vi "Camber controller May 13 2016.vi"() -> ()   [LabVIEW 2014]
uses:
  Environmental Chamber LabVIEW and Instruments/Drivers and Software/keithley_24xx/Keithley 24XX/Keithley 24XX.lvlib
  Environmental Chamber LabVIEW and Instruments/Drivers and Software/keithley_6430/Keithley 6430/Keithley 6430.lvlib
  <vilib>/Instr/_visa.llb/VISA Configure Serial Port (Instr).vi
  <vilib>/Utility/file.llb/Write To Spreadsheet File (string).vi
  Environmental Chamber LabVIEW and Instruments/Drivers and Software/Keithley 2100 Series/Keithley 2100 Series.lvlib
  Environmental Chamber LabVIEW and Instruments/Drivers and Software/Keithley 2100 Series/Public/Configure/Configure 2 Wire Resistance.vi
  Environmental Chamber LabVIEW and Instruments/Drivers and Software/LabVIEW 8.2 Drivers/keithley_24xx/Keithley 24XX/Public/Data/Read (Single Point).vi
  Environmental Chamber LabVIEW and Instruments/Drivers and Software/keithley_6430/Keithley 6430/Public/Data/Read (Single Point).vi
  <vilib>/Utility/file.llb/Read From Spreadsheet File (string).vi
panel:
  out "Cluster":T1
  out "K-2100 (Ohm)":cluster{"Measurement":dbl}(graph)
  out "pressure chart":cluster{"pressure":dbl}(graph)
  out "K-6430 (Ohm)":cluster{"Measurement":dbl}(graph)
  out "K-2420 (Ohm)":cluster{"Resistance":sgl}(graph)
  in  "Data saving options":T2={"Save during sequence only"=TRUE, "Save now"=FALSE, "Stop program when sequence ends"=TRUE, "Delay between data points (s)"=0.0, "Experiment Notes"="", "Currently saving data"=FALSE, "Data file save path"=path ""} {"Delay between data points (s)" min=0.0 max=30.0 format="%#_13g"}
  in  "Set pressure parameters":T3={"valve % open"=100.0, "Desired pressure"=0.0, "Vapor sccm"=0.0, "Gas sccm"=0.0, "Valve"=enum."% Open", "Pressure Mode"=enum."Abs. pressure", "analyte partial pressure"=100.0} {"analyte partial pressure" min=0.0 max=100.0 step=5.0; "Gas sccm" min=0 max=200 step=5; "Vapor sccm" min=0 max=200 step=5; "Desired pressure" min=0.0 max=760.0 step=5.0; "valve % open" min=0.0 max=100.0 step=5.0 format="%#_2f"}
  out "Actual":T4 {"actual gas flow" format="%#_3g"; "Actual vapor flow" format="%#_3g"; "actual pressure" format="%#_3g"; "Valve position (%)" format="%#_2f"}
  out "arduino QCM plots":T5
  out "QCM Freq. (MHz)":T6 {"QCM1" format="%#_8g"; "QCM2" format="%#_8g"; "QCM3" format="%#_8g"; "QCM4" format="%#_8g"; "QCM5" format="%#_8g"; "QCM6" format="%#_8g"}
  in  "Sample names":T7={"QCM1"="aQCM2", "QCM2"="aQCM2", "QCM3"="aQCM3", "QCM4"="aQCM4", "QCM5"="aQCM5", "QCM6"="aQCM6", "SRS"="sample_SRS", "K-2420"="Keithley2420", "K-6430"="Keithley6430", "K-2100"="Keithley6430"}
  out "Sequence\npreview":cluster{dbl[], dbl[]}[](graph)
  in  "Gate time":u16(ring)=1 items=["0.1 seconds", "1.0 seconds", "10.0 seconds"]
  out "MHz":dbl format="%.6f"
  out "QCM plot":T8(graph)
  in  "User-defined\nsequence":string[][](table) caption="Create sequence"
  out "Sequence end time":string
  in  "Run Sequence":bool
  in  "Import sequence file":bool
  in  "Save sequence":bool
  in  "Clear sequence":bool
  in  "Turbo pump\nauto on":bool=TRUE caption="Turbo pump auto on"
  in  "stop":bool
  in  "Clear all charts":bool
  out "appended array":dbl[](array[numeric]) caption="atm\nTorr"
  in  "rapidox O2 Sensor":bool
  in  "setnag O2 Pump":bool
  in  "Baud Rate 2":i32(ring)=2 items=["2400", "4800", "9600", "19200", "38400", "57600", "115200"]
  in  "Com Port":i32(ring) items=["Com 1", "Com 2", "Com 3", "Com 4", "Com 5", "Com 6", "COM 7", "COM 8", "COM 9", "COM 10", "COM 11", "COM 12", "com 13", "COM 14"]
  in  "Com Port 2":i32(ring) items=["Com 1", "Com 2", "Com 3", "Com 4", "Com 5", "Com 6", "COM 7", "COM 8", "COM 9", "COM 10", "COM 11", "COM 12", "com 13", "COM 14"]
  out "Waveform Chart":cluster{dbl}(graph)
  out "O2 Concentration (PPM)":dbl
  out "Waveform Chart 6":cluster{dbl}(graph)
  # "Pressure Control"
  # "Gas/Vapor Sequence"
  # "SRS QCM"
  # "Currently Unused"
  # "100%"
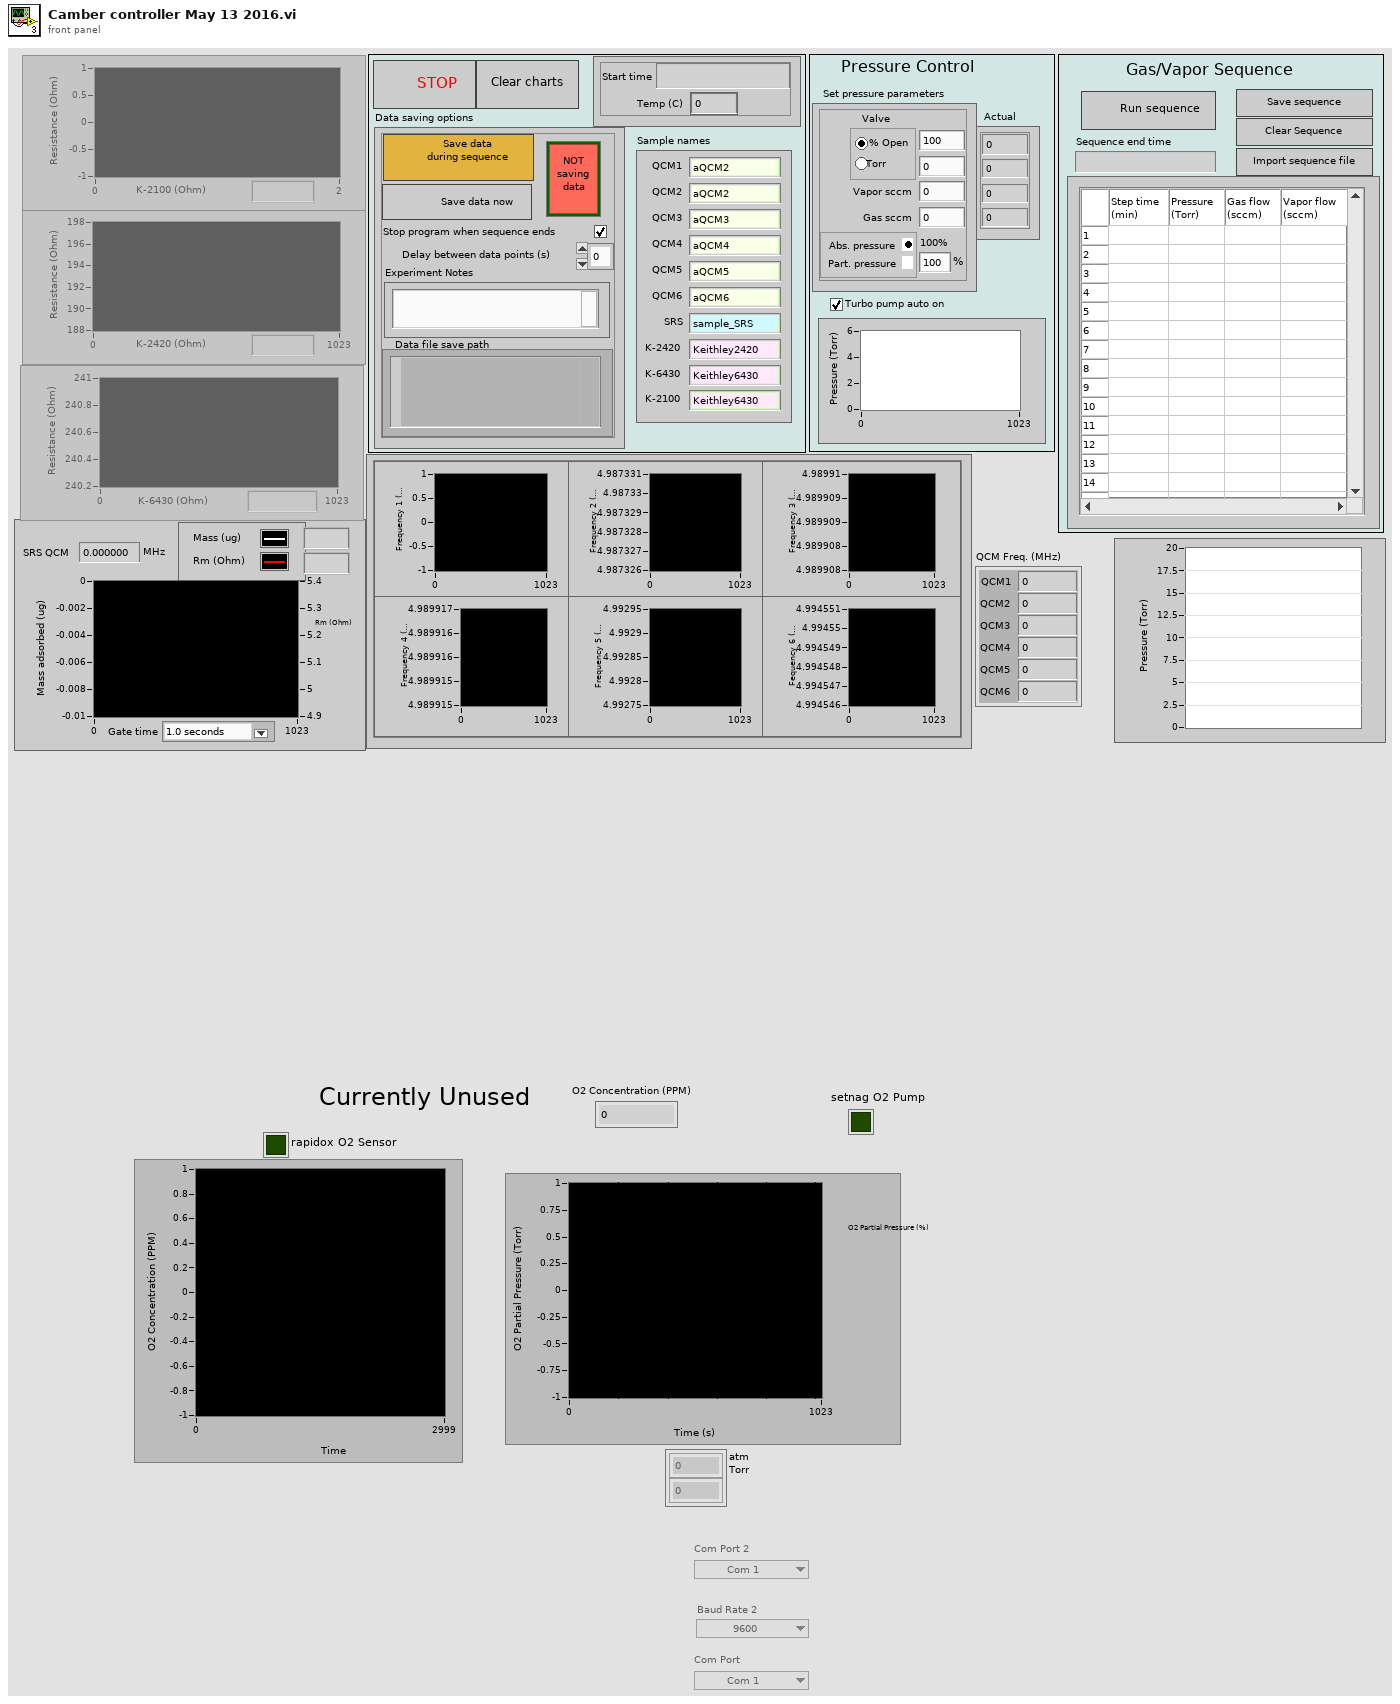
[diagram p1: front panel]
types:
  T1 = cluster{"State date/time":string, "Temp (C)":dbl}
  T2 = cluster{"Save during sequence only":bool, "Save now":bool, "Stop program when sequence ends":bool, "Delay between data points (s)":dbl, "Experiment Notes":string, "Currently saving data":bool, "Data file save path":path}
  T3 = cluster{"valve % open":dbl, "Desired pressure":dbl, "Vapor sccm":sgl, "Gas sccm":sgl, "Valve":enum32{"% Open", "Torr "}, "Pressure Mode":enum32{"Abs. pressure", " Part. pressure"}, "analyte partial pressure":dbl}
  T4 = cluster{"Valve position (%)":dbl, "actual pressure":dbl, "Actual vapor flow":dbl, "actual gas flow":dbl}
  T5 = cluster{"arduino qcm 1":dbl, "arduino qcm 2":dbl, "arduino qcm 3":dbl, "arduino qcm 4":dbl, "arduino qcm 5":dbl, "arduino qcm 6":dbl}
  T6 = cluster{"QCM1":dbl, "QCM2":dbl, "QCM3":dbl, "QCM4":dbl, "QCM5":dbl, "QCM6":dbl}
  T7 = cluster{"QCM1":string, "QCM2":string, "QCM3":string, "QCM4":string, "QCM5":string, "QCM6":string, "SRS":string, "K-2420":string, "K-6430":string, "K-2100":string}
  T8 = cluster{"Numeric Control":dbl, "Resistance out":dbl}
  T9 = enum16{"open", "open or create", "create or replace", "create", "open (read only)"}
  T10 = enum8{"Enabled", "Disabled", "Disabled and Grayed Out"}
  T11 = cluster{"task out":refnum<k21>, "error out":errorcluster, "task out":refnum<k21>, "error out":errorcluster, "task out":refnum<k21>, "error out":errorcluster, "VISA resource name":refnum<visa-resource-name>, "error out":errorcluster}
  T12 = cluster{"task out":refnum<k21>, "error out":errorcluster, "task out":refnum<k21>, "error out":errorcluster, "task out":refnum<k21>, "error out":errorcluster, "VISA resource name out":refnum<visa-resource-name>, "error out":errorcluster}
  T13 = enum16{"no parity", "odd parity", "even parity", "mark parity", "space parity"}
  T14 = cluster{bool, "VISA resource name":refnum<visa-resource-name>, "error out":errorcluster}
  T15 = cluster{bool, "VISA resource name out":refnum<visa-resource-name>, "error out":errorcluster}
  T16 = cluster{"Arduino 1":refnum<visa-resource-name>, "Arduino 2":refnum<visa-resource-name>, "Arduino 3":refnum<visa-resource-name>, "Arduino 4":refnum<visa-resource-name>, "Arduino 5":refnum<visa-resource-name>, "Arduino 6":refnum<visa-resource-name>}
  T17 = cluster{"VISA resource name out":refnum<visa-resource-name>, "error out":errorcluster, "VISA resource name out":refnum<visa-resource-name>, "error out":errorcluster, "VISA resource name out":refnum<visa-resource-name>, "error out":errorcluster, "VISA resource name out":refnum<visa-resource-name>, "error out":errorcluster, "VISA resource name out":refnum<visa-resource-name>, "error out":errorcluster, "VISA resource name out":refnum<visa-resource-name>, "error out":errorcluster}
  T18 = cluster{"f":dbl, "f":dbl, "f":dbl, "f":dbl, "f":dbl, "f":dbl}
  T19 = cluster{"String":string, "String":string, "String":string}
  T20 = cluster{"Boolean":bool, "VISA resource name out":refnum<visa-resource-name>, "error out":errorcluster}
  T21 = cluster{"Numeric Control":dbl, "Cluster":cluster{"Numeric Control":dbl}, "String":string, "error out":errorcluster}
  T22 = cluster{bool, "Turbo pump\nauto on":bool, "current  step # out":i32}
  T23 = cluster{"date/time string":string, "Temp (C)":dbl}
  T24 = cluster{"Present (s)":dbl, "Run Sequence":bool, "Set pressure parameters":cluster{"valve % open":dbl, "Desired pressure":dbl, "Vapor sccm":sgl, "Gas sccm":sgl, "Valve":enum32{"% Open", "Torr "}, "Pressure Mode":enum32{"Abs. pressure", " Part. pressure"}, "analyte partial pressure":dbl}, "sequence end time":timestamp}
  T25 = cluster{"f":dbl, "f":dbl, "f":dbl, "f":dbl, "f":dbl}[]
  T26 = cluster{"VISA Refnum out":refnum<visa-resource-name>, "error out":errorcluster, "VISA Refnum out":refnum<visa-resource-name>, "error out":errorcluster, "VISA Refnum out":refnum<visa-resource-name>, "error out":errorcluster, "VISA Refnum out":refnum<visa-resource-name>, "error out":errorcluster, "VISA Refnum out":refnum<visa-resource-name>, "error out":errorcluster, "VISA Refnum out":refnum<visa-resource-name>, "error out":errorcluster}
  T27 = cluster{"f":string, "f":string, "f":string, "f":string, "f":string, "f":string}
  T28 = cluster{bool, "VISA out":refnum<visa-resource-name>, "error out":errorcluster}
  T29 = cluster{"Boolean":bool, "VISA out":refnum<visa-resource-name>, "error out":errorcluster}
  T30 = cluster{"User-defined\nsequence":refnum<vi>, "Sequence end time":refnum<vi>, "Run Sequence":refnum<vi>}
  T31 = cluster{"pressure":string, "RH":string, "gas flow":string, "vapor flow":string}
  T32 = cluster{"Valve position (%)":dbl, "pressure":dbl, "vapor flow":dbl, "gas flow":dbl}
  T33 = cluster{"task out":refnum<k21>, "error out":errorcluster, "task out":refnum<k21>, "error out":errorcluster, "task out":refnum<k21>, "error out":errorcluster, "VISA Refnum out":refnum<visa-resource-name>, "error out":errorcluster}
  T34 = cluster{"sequence on?":bool, "sequence end time":timestamp, "current  step # out":i32}
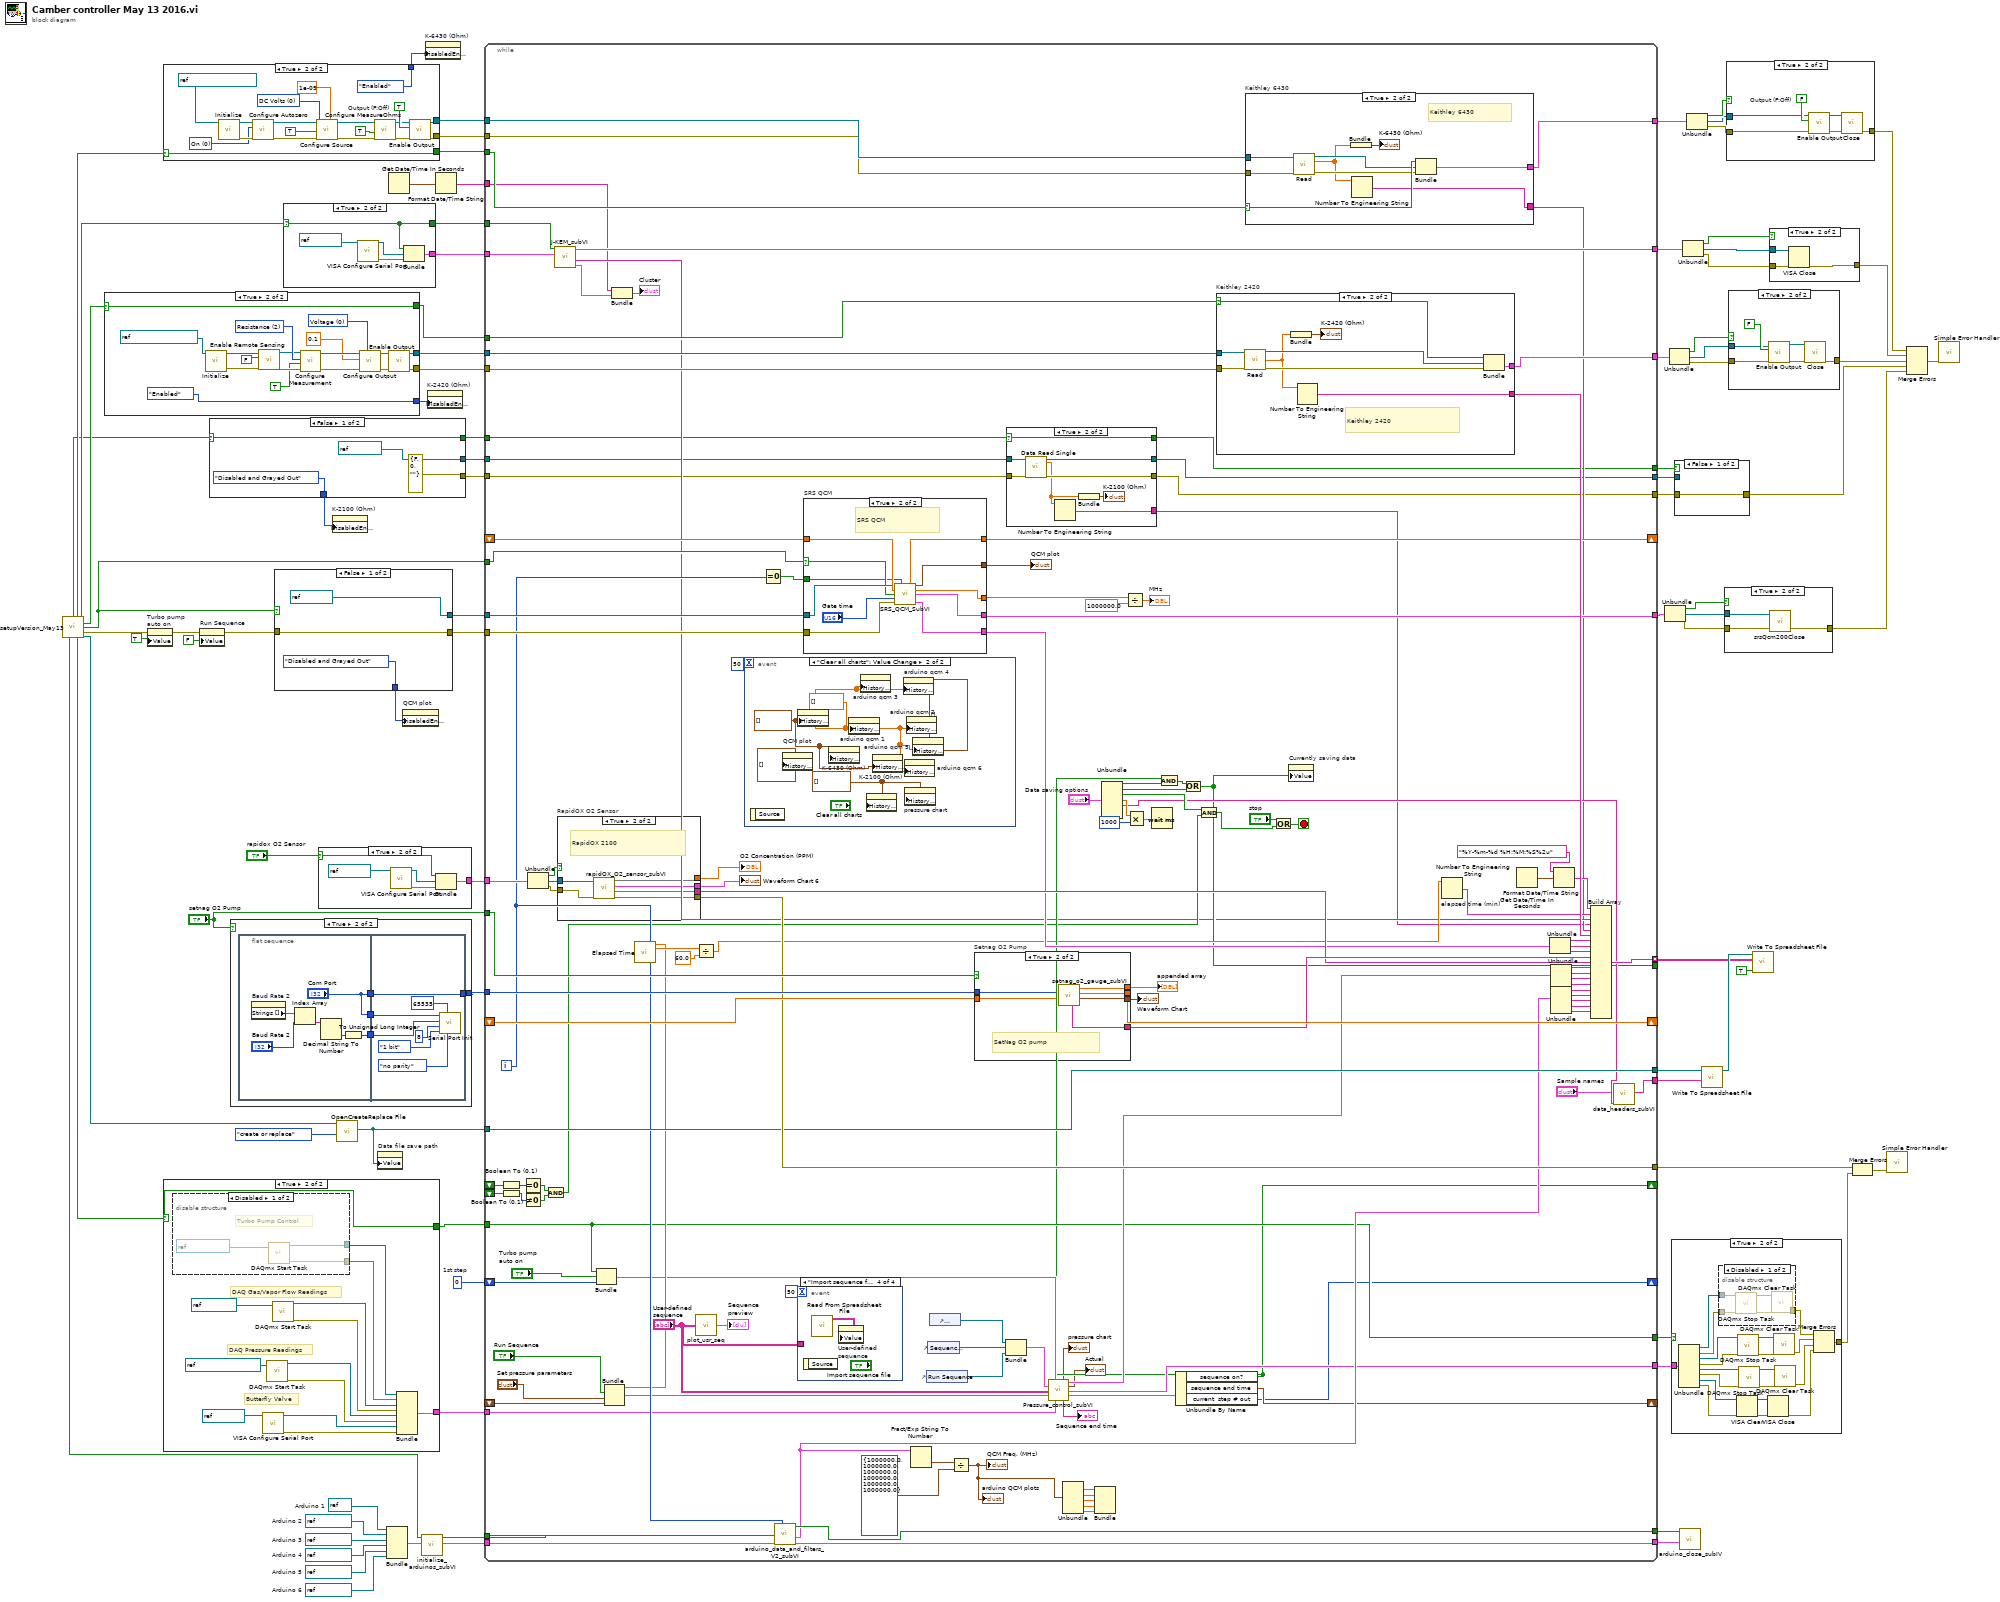
[diagram p0: block diagram]
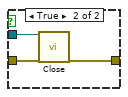
[diagram p2: hidden frame]
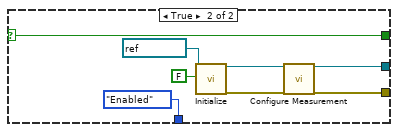
[diagram p3: hidden frame]
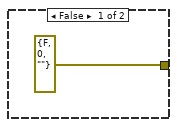
[diagram p4: hidden frame]
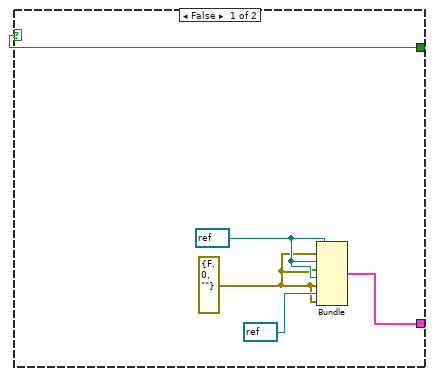
[diagram p6: hidden frame]
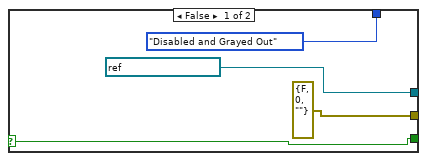
[diagram p9: hidden frame]
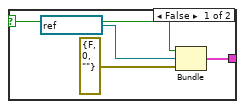
[diagram p10: hidden frame]
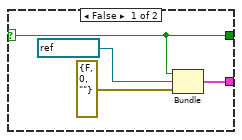
[diagram p12: hidden frame]
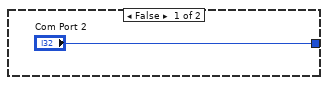
[diagram p13: hidden frame]
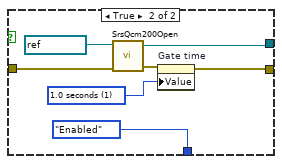
[diagram p15: hidden frame]
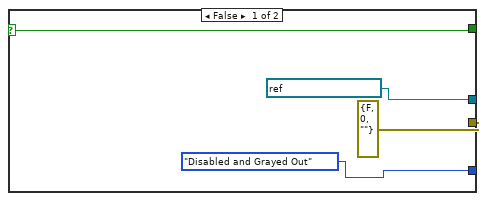
[diagram p17: hidden frame]
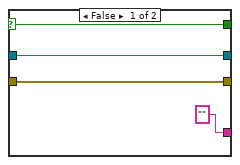
[diagram p18: hidden frame]
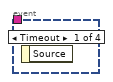
[diagram p19: hidden frame]
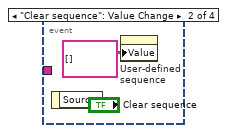
[diagram p20: hidden frame]
diagram:
  w27 = refnum<visa-resource-name> "COM52"  # Arduino 6
  w28 = refnum<visa-resource-name> "COM51"  # Arduino 5
  w29 = refnum<visa-resource-name> "COM50"  # Arduino 4
  w30 = refnum<visa-resource-name> "COM49"  # Arduino 3
  w31 = refnum<visa-resource-name> "COM48"  # Arduino 2
  w20 = refnum<visa-resource-name> refnum  # Arduino 1
  w47 = 0  # 1st step
  n1 = call "setupVersion_May13.vi"() -> ("Keithley 2100 out"=w3:bool, "Keithley 6431"=w37:bool, "J-KEM2"=w36:bool, "Keithley 2421"=w16:bool, "SRS QCM 2"=w40:bool, "error IO"=w12:errorcluster, "Arduino2"=w25:bool, "Pressure control 2"=w38:bool, "Save file path 2"=w39:path)  [unwired: 7 in]
  n2 = case shown="True" w16 {
    selector: w16 -> [w88 w92]
    tunnel: [refnum<visa-resource-name> "GPIB1::24::INSTR" ("VISA resource name") w101] -> w85
    tunnel: [errorcluster {"status"=FALSE, "code"=0, "source"=""} ("error out") w96] -> w84
    tunnel: [T10."Disabled and Grayed Out" ("Disabled") T10."Enabled" ("Disabled")] -> w34
    tunnel: [w88 w92] -> w15
    frame False {
    }
    frame True {
      w103 = u16 0 items=["Voltage", "Current"] ("Source Mode  (0: Voltage)")
      w108 = u16 2 items=["Volts", "Current", "Resistance"] ("Function (0: Volts)")
      n3 = call "Initialize.vi"("VISA resource name"=refnum<visa-resource-name> "GPIB1::24::INSTR") -> ("error out"=w97:errorcluster, "VISA resource name out"=w100:refnum<visa-resource-name>)  [unwired: 9 in]
      n4 = call "Enable Remote Sensing.vi"("error in (no error)"=w97, "Enable Remote Sensing (T: Enable)"=FALSE ("4-wire?"), "VISA resource name"=w100) -> ("error out"=w98:errorcluster, "VISA resource name out"=w99:refnum<visa-resource-name>)  [unwired: 7 in]
      n5 = call "Configure Measurement.vi"("error in (no error)"=w98, "Enable Auto Range (T:Enable)"=TRUE, "Function (0: Volts)"=w108, "VISA resource name"=w99) -> ("error out"=w107:errorcluster, "VISA resource name out"=w106:refnum<visa-resource-name>)  [unwired: 6 in]
      n6 = call "Configure Output.vi"("Source Mode  (0: Voltage)"=w103, "error in (no error)"=w107, "Output Level (0)"=0.1 ("Applied Voltage (V)"), "VISA resource name"=w106) -> ("error out"=w105:errorcluster, "VISA resource name out"=w104:refnum<visa-resource-name>)  [unwired: 6 in]
      n7 = call "Enable Output.vi"("error in (no error)"=w105, "VISA resource name"=w104) -> ("error out"=w96:errorcluster, "VISA resource name out"=w101:refnum<visa-resource-name>)  [unwired: 8 in]
    }
  }
  n8 = property on="Turbo pump\nauto on" class="Bool (strict)"(error in=w12, "Value"=TRUE ("Turbo\npump")) -> (error out=w43:errorcluster)  [unwired: 1 in, 1 out]
  n9 = case shown="True" w37 {
    selector: w37 -> [w110 w114]
    tunnel: [refnum<visa-resource-name> "GPIB0::29::INSTR" ("VISA resource name") w127] -> w54
    tunnel: [errorcluster {"status"=FALSE, "code"=0, "source"=""} ("error out") w128] -> w53
    tunnel: [T10."Disabled and Grayed Out" ("Disabled") T10."Enabled" ("Disabled")] -> w33
    tunnel: [w110 w114] -> w14
    frame False {
    }
    frame True {
      w116 = u16 0 items=["DC Volts", "DC Current"] ("Source Function (0: DC Volts)")
      w123 = u16 0 items=["On", "Off", "Once"] ("Autozero  (0: On)")
      w131 = TRUE  # Output (F:Off)
      n10 = call "Initialize.vi"("VISA resource name"=refnum<visa-resource-name> "GPIB0::30::INSTR") -> ("error out"=w124:errorcluster, "VISA resource name out"=w125:refnum<visa-resource-name>)  [unwired: 4 in, 5 out]
      n11 = call "Configure Autozero.vi"("error in (no error)"=w124, "Autozero  (0: On)"=w123, "VISA resource name"=w125) -> ("error out"=w119:errorcluster, "VISA resource name out"=w121:refnum<visa-resource-name>)  [unwired: 7 in]
      n12 = call "Configure Source.vi"("I-Source Level [A]"=1e-09, "error in (no error)"=w119, "Auto Range (T:Enable)"=TRUE, "Source Function (0: DC Volts)"=w116, "VISA resource name"=w121) -> ("error out"=w118:errorcluster, "VISA resource name out"=w120:refnum<visa-resource-name>)  [unwired: 5 in]
      n13 = call "Configure MeasureOhms.vi"("error in (no error)"=w118, "Auto Range (T:Enable)"=TRUE, "VISA resource name"=w120) -> ("error out"=w132:errorcluster, "VISA resource name out"=w130:refnum<visa-resource-name>)  [unwired: 3 in, 4 out]
      n14 = call "Enable Output.vi"("error in (no error)"=w132, "Enable Output (F:Off)"=w131, "VISA resource name"=w130) -> ("error out"=w128:errorcluster, "VISA resource name out"=w127:refnum<visa-resource-name>)  [unwired: 7 out]
    }
  }
  n15 = case shown="True" w38 {
    selector: w38 -> [w133 w138]
    tunnel: [w134 w140] -> w48
    tunnel: [w133 w138] -> w13
    frame False {
      w136 = refnum<k21> refnum ("task out")
      w135 = errorcluster {"status"=FALSE, "code"=0, "source"=""} ("error out")
      n16 = Bundle("task out"=w136, "error out"=w135, "task out"=w136, "error out"=w135, "task out"=w136, "error out"=w135, "VISA resource name"=refnum<visa-resource-name> refnum, "error out"=w135) -> (w134:T11)  [unwired: 1 in]
    }
    frame True {
      # "DAQ Gas/Vapor Flow Readings"
      # "DAQ Pressure Readings"
      # "Butterfly Valve"
      n17 = disable-structure shown="Disabled" {
        disable-tunnel: [w152 _] -> w147
        disable-tunnel: [w151 _] -> w146
        frame Disabled {
          # "Turbo Pump Control"
          n18 = call <vilib>:"DAQmx Start Task.vi"("task/channels in"=refnum<k21> "TurboON") -> ("task out"=w152:refnum<k21>, "error out"=w151:errorcluster)  [unwired: 13 in]
        }
        frame Enabled {
        }
      }
      n19 = call-poly "VISA Configure Serial Port"("VISA resource name"=refnum<visa-resource-name> "COM5") -> ("VISA resource name out"=w141:refnum<visa-resource-name>, "error out"=w139:errorcluster)  [unwired: 13 in]
      n20 = call <vilib>:"DAQmx Start Task.vi"("task/channels in"=refnum<k21> "AllDaqReadings") -> ("task out"=w143:refnum<k21>, "error out"=w142:errorcluster)  [unwired: 13 in]
      n21 = call <vilib>:"DAQmx Start Task.vi"("task/channels in"=refnum<k21> "Setflow") -> ("task out"=w145:refnum<k21>, "error out"=w144:errorcluster)  [unwired: 13 in]
      n22 = Bundle("task out"=w147, "error out"=w146, "task out"=w145, "error out"=w144, "task out"=w143, "error out"=w142, "VISA resource name out"=w141, "error out"=w139) -> (w140:T12)  [unwired: 1 in]
    }
  }
  n23 = property on="Run Sequence" class="Bool (strict)"(error in=w43, "Value"=FALSE ("Run Sequence")) -> (error out=w45:errorcluster)  [unwired: 1 in, 1 out]
  n24 = case shown="False" w3 {
    selector: w3 -> [w155 w159]
    tunnel: [refnum<visa-resource-name> "K-2100" ("VISA resource name out") w162] -> w10
    tunnel: [errorcluster {"status"=FALSE, "code"=0, "source"=""} ("error out") w161] -> w9
    tunnel: [w155 w159] -> w8
    tunnel: [T10."Disabled and Grayed Out" ("Disabled") T10."Enabled" ("Disabled")] -> w2
    frame False {
    }
    frame True {
      n25 = call "Initialize.vi"("VISA resource name"=refnum<visa-resource-name> "K-2100", "Reset? (T: Reset)"=FALSE) -> ("VISA resource name out"=w163:refnum<visa-resource-name>, "error out"=w160:errorcluster)  [unwired: 16 in]
      n26 = call-poly "Configure Measurement.vi"("VISA resource name"=w163, "error in (no error)"=w160) -> ("VISA resource name out"=w162:refnum<visa-resource-name>, "error out"=w161:errorcluster)  [unwired: 16 in]
    }
  }
  n27 = case shown="True" "setnag O2 Pump" {
    tunnel: ["Com Port 2" w167] -> w81
    frame False {
    }
    frame True {
      n28 = flat-sequence {
        tunnel: ["Com Port"] -> w170
        tunnel: [w172] -> w169
        tunnel: ["Com Port"] -> w168
        tunnel: w170 -> [w178]
        tunnel: w169 -> [w177]
        tunnel: w168 -> [w179]
        tunnel: [w179] -> w167
        frame #0 {
          n29 = property on="Baud Rate 2" class="Ring (strict)"() -> ("Strings []"=w174:string[])  [unwired: 2 in, 2 out]
          n30 = Index Array(array=w174, index="Baud Rate 2") -> (element=w175:string)
          n31 = Decimal String To Number(string=w175) -> (number=w173:i32)  [unwired: 2 in, 1 out]
          n32 = To Unsigned Long Integer(number=w173) -> (unsigned 32bit integer=w172:u32)
        }
        frame #1 {
          n33 = call <vilib>:"Serial Port Init.vi"("parity"=T13."no parity", "buffer size"=u16 65535, "stop bits"=enum16{"1 bit", "1.5 bits", "2 bits"}."1 bit", "data bits"=u16 8, "baud rate"=w177, "port number"=w178) -> ()  [unwired: 1 in, 1 out]
        }
      }
    }
  }
  n34 = case shown="False" w40 {
    tunnel: [refnum<visa-resource-name> "COM6" ("VISA in") w190] -> w83
    tunnel: [w185 w187] -> w82
    tunnel: w45 -> [w185 w192]
    tunnel: [T10."Disabled and Grayed Out" ("Disabled") T10."Enabled" ("Disabled")] -> w35
    frame False {
    }
    frame True {
      w189 = u16 1 items=["0.1 seconds", "1.0 seconds", "10.0 seconds"] ("Gate time")
      n35 = call "SrsQcm200Open.vi"("error in"=w192, "VISA in"=refnum<visa-resource-name> "COM6") -> ("error out"=w188:errorcluster, "VISA out"=w190:refnum<visa-resource-name>)  [unwired: 3 in]
      n36 = property on="Gate time" class="Ring (strict)"(error in=w188, "Value"=w189) -> (error out=w187:errorcluster)  [unwired: 1 in, 1 out]
    }
  }
  n37 = case shown="True" w36 {
    selector: w36 -> [w194 w199]
    tunnel: [w195 w200] -> w70
    tunnel: [w194 w199] -> w64
    frame False {
      n38 = Bundle(w194, "VISA resource name"=refnum<visa-resource-name> "COM3", "error out"=errorcluster {"status"=FALSE, "code"=0, "source"=""}) -> (w195:T14)  [unwired: 1 in]
    }
    frame True {
      n39 = call-poly "VISA Configure Serial Port"("VISA resource name"=refnum<visa-resource-name> "COM3") -> ("VISA resource name out"=w201:refnum<visa-resource-name>, "error out"=w198:errorcluster)  [unwired: 13 in]
      n40 = Bundle(w199, "VISA resource name out"=w201, "error out"=w198) -> (w200:T15)  [unwired: 1 in]
    }
  }
  n41 = case shown="True" "rapidox O2 Sensor" {
    selector: "rapidox O2 Sensor" -> [w203 w208]
    tunnel: [w204 w209] -> w60
    frame False {
      n42 = Bundle(w203, "VISA resource name"=refnum<visa-resource-name> "COM7", "error out"=errorcluster {"status"=FALSE, "code"=0, "source"=""}) -> (w204:T14)  [unwired: 1 in]
    }
    frame True {
      n43 = call-poly "VISA Configure Serial Port"("VISA resource name"=refnum<visa-resource-name> "COM7") -> ("VISA resource name out"=w210:refnum<visa-resource-name>, "error out"=w207:errorcluster)  [unwired: 13 in]
      n44 = Bundle(w208, "VISA resource name out"=w210, "error out"=w207) -> (w209:T15)  [unwired: 1 in]
    }
  }
  n45 = property on="K-2100 (Ohm)" class="WFChart (strict)"("DisabledEnum"=w2) -> ()  [unwired: 2 in, 2 out]
  n46 = call "OpenCreateReplace File.vi"("function (open:0)"=T9."create or replace", "file path"=w39) -> ("new file path"=w11:path)  [unwired: 6 in, 3 out]
  n47 = property on="Data file save path" class="Path"("Value"=w11) -> ()  [unwired: 2 in, 2 out]
  n48 = Bundle("Arduino 1"=w20, "Arduino 2"=w31, "Arduino 3"=w30, "Arduino 4"=w29, "Arduino 5"=w28, "Arduino 6"=w27) -> (w19:T16)  [unwired: 1 in]
  n49 = Get Date/Time In Seconds() -> (seconds since 1Jan1904=w87:timestamp)
  n50 = property on="QCM plot" class="WFChart (strict)"("DisabledEnum"=w35) -> ()  [unwired: 2 in, 2 out]
  n51 = call "initialize_arduinos_subVI.vi"("arduino 1-6 addresses"=w19, "arduinos on?"=w25) -> ("arduino 1-6 address and errors"=w24:T17, "arduinos on/off"=w26:bool)  [unwired: 8 in]
  n52 = property on="K-6430 (Ohm)" class="WFChart (strict)"("DisabledEnum"=w33) -> ()  [unwired: 2 in, 2 out]
  n53 = property on="K-2420 (Ohm)" class="WFChart (strict)"("DisabledEnum"=w34) -> ()  [unwired: 2 in, 2 out]
  n54 = Format Date/Time String(seconds (now)=w87) -> (date/time string=w1:string)  [unwired: 2 in]
  n55 = while {
    shift-right: [w346] -> _
    shift-left: _ -> [w345]
    tunnel: [w317] -> w32 mode=indexing if=w231
    tunnel: w15 -> [w323]
    tunnel: w85 -> [w344]
    tunnel: w84 -> [w343]
    tunnel: w83 -> [w342]
    tunnel: w82 -> [w341]
    tunnel: w40 -> [w340]
    tunnel: "setnag O2 Pump" -> [w334]
    tunnel: w81 -> [w339]
    tunnel: [w336] -> w78
    tunnel: [w335] -> w74
    tunnel: w70 -> [w333]
    tunnel: [w332] -> w69
    tunnel: w64 -> [w331]
    tunnel: w60 -> [w329]
    tunnel: [w324] -> w41
    tunnel: [w322] -> w59
    tunnel: w11 -> [w322]
    shift-right: [w315] -> _
    shift-left: _ -> [w316]
    tunnel: w54 -> [w321]
    tunnel: w53 -> [w320]
    tunnel: [w319] -> w52
    tunnel: w13 -> [w262]
    tunnel: [w262] -> w49
    tunnel: w48 -> [w256]
    shift-right: [w258] -> _
    shift-left: w47 -> [w264]
    tunnel: [w231] -> _
    shift-right: [w259] -> _
    shift-left: _ -> [w273]
    tunnel: w26 -> [w300]
    tunnel: w24 -> [w299]
    tunnel: [w298] -> w22
    tunnel: [w297] -> w23
    tunnel: [w288] -> w21
    tunnel: [w275] -> w18
    tunnel: w14 -> [w274]
    shift-right: [w242] -> _
    shift-left: _ -> [w254]
    shift-left: _ -> [w253]
    tunnel: w10 -> [w227]
    tunnel: w9 -> [w226]
    tunnel: w8 -> [w224]
    tunnel: [w223] -> w7
    tunnel: [w222] -> w6
    tunnel: [w221] -> w5
    tunnel: w1 -> [w213]
    i -> [w301]
    stop <- w238 stop-if-true
    n56 = Boolean To (0,1)(Boolean=w254) -> (0, 1=w252:i16)
    n57 = Boolean To (0,1)(Boolean=w253) -> (0, 1=w251:i16)
    n58 = Equal To 0?(x=w252) -> (x = 0?=w249:bool)
    n59 = Not Equal To 0?(x=w251) -> (x != 0?=w250:bool)
    n60 = Unbundle(w329) -> (w328:bool, "VISA resource name out"=w327:refnum<visa-resource-name>, "error out"=w326:errorcluster)
    n61 = And(x=w249, y=w250) -> (x .and. y?=w236:bool)
    n62 = call "J-KEM_subVI.vi"("Address in"=w333, "J-KEM on?"=w331) -> ("Temp (C)"=w212:dbl, "String data out"=w229:string, "Address out"=w332:T20)  [unwired: 6 in, 1 out]
    n63 = case "RapidOX O2 Sensor" shown="True" w328 {
      tunnel: w327 -> [_ w390]
      tunnel: w326 -> [w383 w389]
      tunnel: ["" w388] -> w325
      tunnel: [w383 w387] -> w324
      tunnel: [0.0 w386] -> w313
      tunnel: [cluster{dbl} {0.0} w385] -> w312
      frame False {
      }
      frame True {
        # "RapidOX 2100"
        n64 = call "rapidOX_O2_sensor_subVI.vi"(8:w389, 11:w390) -> (0:w387, 1:w388, "rapidox info out"=w385:T21, 3:w386)  [unwired: 6 in]
      }
    }
    "O2 Concentration (PPM)" <- w313
    "Waveform Chart 6" <- w312
    n65 = Bundle(w262, "Turbo pump\nauto on"="Turbo pump\nauto on", "current  step # out"=w264) -> (w261:T22)  [unwired: 1 in]
    n66 = Bundle("date/time string"=w213, "Temp (C)"=w212) -> (→"Cluster":T23)  [unwired: 1 in]
    n67 = call "Elapsed Time"() -> ("Present (s)"=w282:dbl, "Elapsed Time (s)"=w314:dbl)  [unwired: 12 in, 6 out]
    n68 = Bundle("Present (s)"=w282, "Run Sequence"="Run Sequence", "Set pressure parameters"="Set pressure parameters", "sequence end time"=w273) -> (w255:T24)  [unwired: 1 in]
    n69 = Divide(x=w314, y=60.0) -> (x/y=w240:dbl)
    n70 = call "plot_usr_seq.vi"("User-defined sequence"="User-defined\nsequence") -> ("Sequence Preview"=→"Sequence\npreview":cluster{dbl[], dbl[]}[])
    n71 = event shown="[1] \"Clear all charts\": Value Change" {
      selector: _ -> [_ _]
      dyn-events: _ -> [_ _]
      timeout: 50 -> [_ _]
      event Timeout {
        n72 = event-data() -> ()  [unwired: 1 in, 3 out]
      }
      event "Clear all charts": Value Change {
        (unwired) T25 [] ("History Data")
        w364 = cluster{dbl}[] [] ("History Data")
        w363 = cluster{"Resistance":sgl}[] [] ("History Data")
        w365 = dbl[] [] ("History Data")
        n73 = event-data() -> ()  [unwired: 1 in, 1 out]
        n74 = property on="QCM plot" class="WFChart (strict)"("History Data"=cluster{dbl, "Resistance out":dbl}[] []) -> ()  [unwired: 2 in, 2 out]
        n75 = property on="K-2420 (Ohm)" class="WFChart (strict)"("History Data"=w363) -> ()  [unwired: 2 in, 2 out]
        n76 = property on="K-6430 (Ohm)" class="WFChart (strict)"("History Data"=w363) -> ()  [unwired: 2 in, 2 out]
        n77 = property on="arduino qcm 1" class="WFChart (strict)"("History Data"=w365) -> ()  [unwired: 2 in, 2 out]
        n78 = property on="arduino qcm 3" class="WFChart (strict)"("History Data"=w365) -> ()  [unwired: 2 in, 2 out]
        n79 = property on="Waveform Chart" class="WFChart (strict)"("History Data"=w364) -> ()  [unwired: 2 in, 2 out]
        n80 = property on="K-2100 (Ohm)" class="WFChart (strict)"("History Data"=w363) -> ()  [unwired: 2 in, 2 out]
        n81 = property on="arduino qcm 4" class="WFChart (strict)"("History Data"=w365) -> ()  [unwired: 2 in, 2 out]
        n82 = property on="arduino qcm 6" class="WFChart (strict)"("History Data"=w365) -> ()  [unwired: 2 in, 2 out]
        n83 = property on="pressure chart" class="WFChart (strict)"("History Data"=w364) -> ()  [unwired: 2 in, 2 out]
        n84 = property on="arduino qcm 2" class="WFChart (strict)"("History Data"=w365) -> ()  [unwired: 2 in, 2 out]
        n85 = property on="arduino qcm 5" class="WFChart (strict)"("History Data"=w365) -> ()  [unwired: 2 in, 2 out]
      }
    }
    n86 = Equal To 0?(x=w301) -> (x = 0?=w307:bool)
    n87 = call "arduino_data_and_filters_V2_subVI.vi"("loop iteration number"=w301, "arduino 1-6 address and errors"=w299, "arduinos on?"=w300) -> ("arduino 1-6 addresses and errors out"=w297:T26, "arduino 1-6 data out"=w296:T27, "arduinos on? output"=w298:bool)  [unwired: 6 in]
    n88 = event shown="[3] \"Import sequence file\": Value Change" {
      selector: _ -> [_ _ _ _]
      dyn-events: _ -> [_ _ _ _]
      timeout: 50 -> [_ _ _ _]
      tunnel: "User-defined\nsequence" -> [_ _ w361 _]
      event Timeout {
        n89 = event-data() -> ()  [unwired: 1 in, 1 out]
      }
      event "Clear sequence": Value Change {
        n90 = event-data() -> ()  [unwired: 1 in, 1 out]
        n91 = property on="User-defined\nsequence" class="Tbl (strict)"("Value"=string[][] []) -> ()  [unwired: 2 in, 2 out]
      }
      event "Save sequence": Value Change {
        n92 = event-data() -> ()  [unwired: 1 in, 1 out]
        n93 = call-poly <vilib>:"Write To Spreadsheet File.vi"("2D data"=w361) -> ()  [unwired: 7 in, 1 out]
      }
      event "Import sequence file": Value Change {
        n94 = event-data() -> ()  [unwired: 1 in, 1 out]
        n95 = call-poly <vilib>:"Read From Spreadsheet File.vi"() -> ("all rows"=w362:string[][])  [unwired: 7 in, 4 out]
        n96 = property on="User-defined\nsequence" class="Tbl (strict)"("Value"=w362) -> ()  [unwired: 2 in, 2 out]
      }
    }
    n97 = case "SRS QCM" shown="True" w340 {
      selector: w340 -> [w408 w414]
      tunnel: w342 -> [w411 w418]
      tunnel: w341 -> [w410 w419]
      tunnel: [w409 w422] -> w335
      tunnel: w316 -> [_ w421]
      tunnel: [w406 w420] -> w315
      tunnel: [T8 {"Numeric Control"=0.0, "Resistance out"=0.0} ("Cluster") w416] -> w311
      tunnel: [w406 w415] -> w287
      tunnel: w307 -> [_ w413]
      tunnel: [T19 {"String"="", "String"="", "String"=""} ("M,F,MR output cluster") w412] -> w295
      frame False {
        w406 = 0.0
        n98 = Bundle(w408, "VISA out"=w411, "error out"=w410) -> (w409:T28)  [unwired: 1 in]
      }
      frame True {
        # "SRS QCM"
        n99 = call "SRS_QCM_SubVI.vi"("VISA Refnum in"=w418, "first iteration?"=w413, "Frequency out 3"=w421, "Boolean 2"=w414, "Gate time"="Gate time", "error in (no error)"=w419) -> ("Frequency out 2"=w420:dbl, "Cluster"=w416:T8, "Frequency out"=w415:dbl, "Cluster 2"=w422:T29, "M,F,MR output cluster"=w412:T19)  [unwired: 2 in, 3 out]
      }
    }
    "QCM plot" <- w311
    n100 = Fract/Exp String To Number(string=w296) -> (number=w284:T18)  [unwired: 3 in, 1 out]
    n101 = control-ref of="Run Sequence"() -> (w266:refnum<vi>)
    n102 = control-ref of="Sequence end time"() -> (w267:refnum<vi>)
    n103 = control-ref of="User-defined\nsequence"() -> (w268:refnum<vi>)
    n104 = Divide(x=w284, y=T18 {"f"=1000000.0, "f"=1000000.0, "f"=1000000.0, "f"=1000000.0, "f"=1000000.0, "f"=1000000.0}) -> (x/y=w220:T18)
    "QCM Freq. (MHz)" <- w220
    "arduino QCM plots" <- w220
    n105 = case "Setnag O2 Pump" shown="True" w334 {
      tunnel: [w426 w431] -> w346
      tunnel: w345 -> [w426 w432]
      tunnel: w339 -> [_ w430]
      tunnel: ["" w429] -> w338
      tunnel: [dbl[] [] w428] -> w310
      tunnel: [cluster{dbl} {0.0} w427] -> w309
      frame False {
      }
      frame True {
        # "SetNag O2 pump"
        n106 = call "setnag_o2_gauge_subVI.vi"("Numeric Control 3"=w432, "Com Port"=w430) -> ("Cluster"=w427:cluster{"Numeric Control":dbl}, "Numeric Control out"=w431:dbl, "Array"=w428:dbl[], "String"=w429:string)  [unwired: 6 in]
      }
    }
    "appended array" <- w310
    "Waveform Chart" <- w309
    n107 = Bundle("User-defined\nsequence"=w268, "Sequence end time"=w267, "Run Sequence"=w266) -> (w265:T30)  [unwired: 1 in]
    n108 = case shown="True" w224 {
      selector: w224 -> [w348 w352]
      tunnel: [w349 w359] -> w222
      tunnel: [w350 w358] -> w221
      tunnel: w227 -> [w349 w357]
      tunnel: w226 -> [w350 w356]
      tunnel: ["" w354] -> w225
      tunnel: [w348 w352] -> w223
      frame False {
      }
      frame True {
        n109 = call "Data Read Single.vi"("VISA resource name"=w357, "error in (no error)"=w356) -> ("VISA resource name out"=w359:refnum<visa-resource-name>, "Measurement"=w355:dbl, "error out"=w358:errorcluster)  [unwired: 15 in]
        n110 = Number To Engineering String ("elapsed time (min)")(4:w355) -> (0:w354:string)  [unwired: 3 in]
        n111 = Bundle("Measurement"=w355) -> (→"K-2100 (Ohm)":cluster{"Measurement":dbl})  [unwired: 1 in]
      }
    }
    n112 = call "Pressure_control_subVI.vi"("press control on / turb pump on / step #"=w261, "references in"=w265, "User-defined\nsequence"="User-defined\nsequence", "output cluster"=w255, "DAQ IDs in"=w256) -> ("pressure"=→"pressure chart":cluster{"pressure":dbl}, "press/RH/gas/vapor"=w280:T31, "pressure params out"=→"Actual":T32, "DAQ IDs out"=w275:T33, "seq on/timestamp/step#"=w260:T34, "date/time string"=→"Sequence end time":string)  [unwired: 5 in]
    n113 = Unbundle(w220) -> ("f"=w219:dbl, "f"=w218:dbl, "f"=w217:dbl, "f"=w216:dbl, "f"=w215:dbl)  [unwired: 1 out]
    n114 = Bundle("f"=w219, "f"=w218, "f"=w217, "f"=w216, "f"=w215) -> ()  [unwired: 1 in, 1 out]
    n115 = Unbundle("Data saving options") -> ("Save during sequence only"=w243:bool, "Save now"=w246:bool, "Stop program when sequence ends"=w237:bool, "Delay between data points (s)"=w244:dbl, "Experiment Notes"=w234:string)  [unwired: 2 out]
    n116 = Divide(x=w287, y=1000000.0) -> (x/y=→"MHz":dbl)
    n117 = Multiply(x=w244, y=u32 1000 ("x")) -> (x*y=w308:dbl)
    n118 = Wait (ms)(milliseconds to wait=w308) -> ()  [unwired: 1 out]
    n119 = Unbundle By Name(w260) -> ("sequence on?"=w242:bool, "sequence end time"=w259:timestamp, "current  step # out"=w258:i32)
    n120 = And(x=w242, y=w243) -> (x .and. y?=w241:bool)
    n121 = Or(x=w241, y=w246) -> (x .or. y?=w231:bool)
    n122 = And(x=w237, y=w236) -> (x .and. y?=w235:bool)
    n123 = case "Keithley 2420" shown="True" w323 {
      selector: w323 -> [w394 w402]
      tunnel: w344 -> [w393 w397]
      tunnel: w343 -> [w392 w396]
      tunnel: [w391 w400] -> w336
      tunnel: ["" w399] -> w337
      frame False {
        n124 = Bundle(w394, "VISA resource name out"=w393, "error out"=w392) -> (w391:T15)  [unwired: 1 in]
      }
      frame True {
        # "Keithley 2420"
        n125 = call-poly "Read.vi"("VISA resource name"=w397, "error in (no error)"=w396) -> ("VISA resource name out"=w403:refnum<visa-resource-name>, "Resistance"=w398:sgl, "error out"=w401:errorcluster)  [unwired: 7 in, 4 out]
        n126 = Bundle("Resistance"=w398) -> (→"K-2420 (Ohm)":cluster{"Resistance":sgl})  [unwired: 1 in]
        n127 = Number To Engineering String(4:w398) -> (0:w399:string)  [unwired: 3 in]
        n128 = Bundle(w402, "VISA resource name out"=w403, "error out"=w401) -> (w400:T15)  [unwired: 1 in]
      }
    }
    n129 = case "Keithley 6430" shown="True" w274 {
      selector: w274 -> [w370 w380]
      tunnel: w321 -> [w369 w377]
      tunnel: w320 -> [w368 w376]
      tunnel: ["" w379] -> w228
      tunnel: [w367 w378] -> w319
      frame False {
        n130 = Bundle(w370, "VISA resource name out"=w369, "error out"=w368) -> (w367:T15)  [unwired: 1 in]
      }
      frame True {
        # "Keithley 6430"
        n131 = call-poly "Read.vi"("error in (no error)"=w376, "VISA resource name"=w377) -> ("error out"=w375:errorcluster, "Measurement"=w373:dbl, "VISA resource name out"=w374:refnum<visa-resource-name>)  [unwired: 1 in, 6 out]
        n132 = Bundle("Measurement"=w373) -> (→"K-6430 (Ohm)":cluster{"Measurement":dbl})  [unwired: 1 in]
        n133 = Number To Engineering String(4:w373) -> (0:w379:string)  [unwired: 3 in]
        n134 = Bundle(w380, "VISA resource name out"=w374, "error out"=w375) -> (w378:T15)  [unwired: 1 in]
      }
    }
    n135 = Or(x="stop", y=w235) -> (x .or. y?=w238:bool)
    n136 = property on="Currently saving data" class="Bool (strict)"("Value"=w231) -> ()  [unwired: 2 in, 2 out]
    n137 = Number To Engineering String "elapsed time (min)"(4:w240) -> (0:w247:string)  [unwired: 3 in]
    n138 = Get Date/Time In Seconds() -> (seconds since 1Jan1904=w347:timestamp)
    n139 = Unbundle(w295) -> ("String"=w305:string, "String"=w304:string, "String"=w303:string)
    n140 = Unbundle(w280) -> ("pressure"=w279:string, "RH"=w278:string, "gas flow"=w277:string, "vapor flow"=w276:string)
    n141 = Unbundle ("arduino 1-6")(w296) -> ("f"=w294:string, "f"=w293:string, "f"=w292:string, "f"=w291:string, "f"=w290:string, "f"=w289:string)
    n142 = Format Date/Time String(time format string (%c)="%Y-%m-%d %H:%M:%S%2u", seconds (now)=w347) -> (date/time string=w302:string)  [unwired: 1 in]
    n143 = Build Array(w302, w247, w229, w225, w228, w337, w305, w304, w303, w338, w325, w279, w278, w277, w276, w294, w293, w292, w291, w290, w289) -> (w317:string[])
    n144 = call "data_headers_subVI.vi"("Experiment Notes"=w234, "Sample names"="Sample names") -> ("data headers"=w288:string[])  [unwired: 9 in]
  }
  n145 = Unbundle(w74) -> ("Boolean"=w73:bool, "VISA out"=w72:refnum<visa-resource-name>, "error out"=w71:errorcluster)
  n146 = Unbundle(w78) -> (w77:bool, "VISA resource name out"=w76:refnum<visa-resource-name>, "error out"=w75:errorcluster)
  n147 = case shown="True" w49 {
    tunnel: w18 -> [_ w447]
    tunnel: [errorcluster {"status"=FALSE, "code"=0, "source"=""} ("error out") w434] -> w17
    frame False {
    }
    frame True {
      n148 = Unbundle(w447) -> ("task out"=w446:refnum<k21>, "error out"=w445:errorcluster, "task out"=w444:refnum<k21>, "error out"=w443:errorcluster, "task out"=w442:refnum<k21>, "error out"=w441:errorcluster, "VISA Refnum out"=w440:refnum<visa-resource-name>, "error out"=w439:errorcluster)
      n149 = disable-structure shown="Disabled" {
        disable-tunnel: [w456 _] -> w438
        disable-tunnel: w446 -> [w455 _]
        disable-tunnel: w445 -> [w454 _]
        frame Disabled {
          n150 = call <vilib>:"DAQmx Stop Task.vi"("task/channels in"=w455, "error in"=w454) -> ("task out"=w457:refnum<k21>, "error out"=w458:errorcluster)  [unwired: 12 in]
          n151 = call <vilib>:"DAQmx Clear Task.vi"("task in"=w457, "error in"=w458) -> ("error out"=w456:errorcluster)  [unwired: 13 in]
        }
        frame Enabled {
        }
      }
      n152 = VISA Clear(VISA resource name=w440, error in (no error)=w439) -> (VISA resource name out=w449:refnum<visa-resource-name>, error out=w448:errorcluster)
      n153 = call <vilib>:"DAQmx Stop Task.vi"("task/channels in"=w444, "error in"=w443) -> ("task out"=w451:refnum<k21>, "error out"=w450:errorcluster)  [unwired: 12 in]
      n154 = call <vilib>:"DAQmx Stop Task.vi"("task/channels in"=w442, "error in"=w441) -> ("task out"=w452:refnum<k21>, "error out"=w453:errorcluster)  [unwired: 12 in]
      n155 = VISA Close(VISA resource name=w449, error in (no error)=w448) -> (error out=w435:errorcluster)
      n156 = call <vilib>:"DAQmx Clear Task.vi"("task in"=w451, "error in"=w450) -> ("error out"=w437:errorcluster)  [unwired: 13 in]
      n157 = call <vilib>:"DAQmx Clear Task.vi"("task in"=w452, "error in"=w453) -> ("error out"=w436:errorcluster)  [unwired: 13 in]
      n158 = Merge Errors(w438, w437, w436, w435) -> (w434:errorcluster)
    }
  }
  n159 = case shown="False" w7 {
    tunnel: w6 -> [_ w462]
    tunnel: w5 -> [w459 w461]
    tunnel: [w459 w460] -> w4
    frame False {
    }
    frame True {
      n160 = call "Close.vi"("VISA resource name"=w462, "error in (no error)"=w461) -> ("error out"=w460:errorcluster)  [unwired: 17 in]
    }
  }
  n161 = call "arduino_close_subIV.vi"("arduino 1-6 addresses and errors out"=w23, "arduinos on?"=w22) -> ()  [unwired: 10 in]
  n162 = Unbundle(w69) -> ("Boolean"=w68:bool, "VISA resource name out"=w67:refnum<visa-resource-name>, "error out"=w66:errorcluster)
  n163 = Unbundle(w52) -> (w57:bool, "VISA resource name out"=w56:refnum<visa-resource-name>, "error out"=w55:errorcluster)
  n164 = call-poly <vilib>:"Write To Spreadsheet File.vi"("1D data"=w21, "file path (dialog if empty)"=w59) -> ("new file path (Not A Path if cancelled)"=w63:path)  [unwired: 6 in]
  n165 = case shown="True" w73 {
    tunnel: w71 -> [w463 w466]
    tunnel: [w463 w465] -> w80
    tunnel: w72 -> [_ w464]
    frame False {
    }
    frame True {
      n166 = call "srsQcm200Close.vi"("error in"=w466, "Visa in"=w464) -> ("error out"=w465:errorcluster)  [unwired: 3 in]
    }
  }
  n167 = case shown="True" w57 {
    tunnel: w56 -> [_ w469]
    tunnel: w55 -> [w467 w468]
    tunnel: [w467 w470] -> w51
    frame False {
    }
    frame True {
      w473 = FALSE  # Output (F:Off)
      n168 = call "Enable Output.vi"("error in (no error)"=w468, "Enable Output (F:Off)"=w473, "VISA resource name"=w469) -> ("error out"=w471:errorcluster, "VISA resource name out"=w472:refnum<visa-resource-name>)  [unwired: 7 out]
      n169 = call "Close.vi"("error in (no error)"=w471, "VISA resource name"=w472) -> ("error out"=w470:errorcluster)  [unwired: 9 out]
    }
  }
  n170 = case shown="True" w77 {
    tunnel: w76 -> [_ w477]
    tunnel: w75 -> [w474 w476]
    tunnel: [w474 w475] -> w79
    frame False {
    }
    frame True {
      n171 = call "Enable Output.vi"("error in (no error)"=w476, "Enable Output (T: Enable)"=FALSE, "VISA resource name"=w477) -> ("error out"=w478:errorcluster, "VISA resource name out"=w480:refnum<visa-resource-name>)  [unwired: 7 in]
      n172 = call "Close.vi"("error in (no error)"=w478, "VISA resource name"=w480) -> ("error out"=w475:errorcluster)  [unwired: 9 in]
    }
  }
  n173 = call-poly <vilib>:"Write To Spreadsheet File.vi"("append to file? (new file:F)"=TRUE, "2D data"=w32, "file path (dialog if empty)"=w63) -> ()  [unwired: 5 in, 1 out]
  n174 = case shown="True" w68 {
    tunnel: w67 -> [_ w484]
    tunnel: w66 -> [w481 w483]
    tunnel: [w481 w482] -> w65
    frame False {
    }
    frame True {
      n175 = VISA Close(VISA resource name=w484, error in (no error)=w483) -> (error out=w482:errorcluster)
    }
  }
  n176 = Merge Errors(w41, w17) -> (w42:errorcluster)
  n177 = call <vilib>:"Simple Error Handler.vi"("error in (no error)"=w42) -> ()  [unwired: 4 in, 5 out]
  n178 = Merge Errors(w51, w65, w79, w4, w80) -> (w86:errorcluster)
  n179 = call <vilib>:"Simple Error Handler.vi"("error in (no error)"=w86) -> ()  [unwired: 4 in, 5 out]
